vi "ADU.vi"(0 "从设备编号":u8 format="%02x", 1 "ASCII？":bool=TRUE, 5 "功能码":u8(ring)=1 items=["01"=1, "02"=2, "03"=3, "04"=4, "05"=5, "06"=6, "0F"=21, "10"=22], 7 "起始地址":u16 format="%04x", 9 "数据量":u16 format="%04x", 11 "字节数":u16 format="%04x", 12 "数据域":u8[](array[numeric]) format="%04x", 13 "字节数？":bool=TRUE) -> (4 "RTU数据帧":u8[](array[numeric]) format="%02x", 6 "ASCII数据帧":string, 10 "CRC-16":u16 format="%04x", 15 "LRC-8":string)   [LabVIEW 2015]
doc: "应用数据单元数据处理\nCRC-16: CRC校验字符数组，输出已做高低位转置，高位在后 [ Lo, Hi ]。\nLRC-8 : LRC校验字符串，两字节数组，高位在前\n字节数？:true 将包含字节数输入，false将不包含字节数输入"
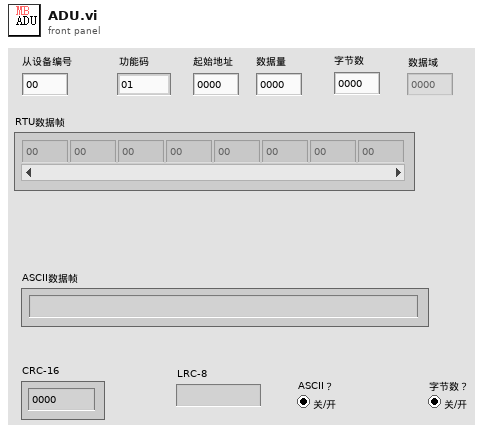
[diagram p1: front panel]
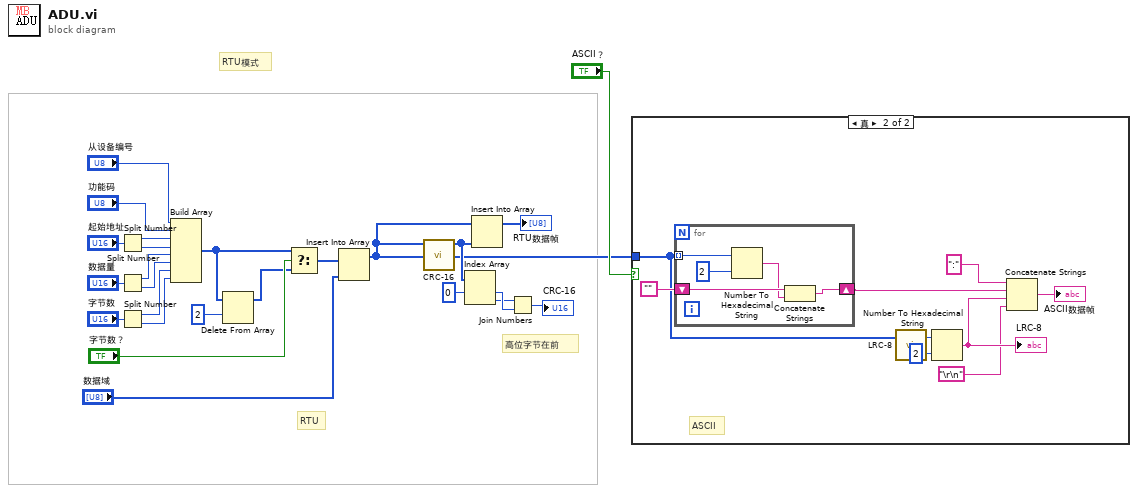
[diagram p0: block diagram]
diagram:
  # "RTU模式"
  # "高位字节在前"
  # "RTU"
  n1 = Split Number(x="起始地址") -> (hi(x)=w22:u8, lo(x)=w21:u8)
  n2 = Split Number(x="数据量") -> (hi(x)=w19:u8, lo(x)=w18:u8)
  n3 = Split Number(x="字节数") -> (hi(x)=w9:u8, lo(x)=w8:u8)
  n4 = Build Array("从设备编号", "功能码", w22, w21, w19, w18, w9, w8) -> (w6:u8[])
  n5 = Delete From Array(array=w6, length=2) -> (array with subset deleted=w4:u8[])  [unwired: 1 in, 1 out]
  n6 = Select(t=w6, s="字节数？", f=w4) -> (s? t:f=w3:u8[])
  n7 = Insert Into Array(array=w3, new element="数据域") -> (w1:u8[])  [unwired: 1 in]
  n8 = call "CRC-16.vi"("Frame in"=w1) -> ("CRC-16"=w16:u8[])  [unwired: 6 in]
  n9 = Index Array(array=w16, index #1=0) -> (element #1=w13:u8, element #2=w12:u8)  [unwired: 1 in]
  n10 = Insert Into Array(array=w1, new element=w16) -> (→"RTU数据帧":u8[])  [unwired: 1 in]
  n11 = Join Numbers(hi=w12, lo=w13) -> ((hi.lo)=→"CRC-16":u16)
  n12 = case shown="真" "ASCII？" {
    tunnel: w1 -> [_ w26]
    frame False {
    }
    frame True {
      # "ASCII"
      n13 = for {
        tunnel: w26 -> [w39] mode=indexing
        shift-right: [w38] -> w30
        shift-left: "" -> [w37]
        n14 = Number To Hexadecimal String(1:2, 2:w39) -> (0:w36:string)
        n15 = Concatenate Strings(w37, w36) -> (w38:string)
      }
      n16 = call "LRC-8.vi"("Frame in"=w26) -> ("LRC-8"=w33:u8)  [unwired: 2 in]
      n17 = Number To Hexadecimal String(1:2, 2:w33) -> (0:w31:string)
      "LRC-8" <- w31
      n18 = Concatenate Strings(":", w30, w31, "\r\n") -> (→"ASCII数据帧":string)
    }
  }
